vi "onPlay.vi"(8 "error in (no error)":errorcluster, 10 "Player In":refnum<class "Player.lvclass">, 11 "ReadyState in":refnum<class "ReadyState.lvclass">) -> (0 "error out":errorcluster, 1 "String":string, 2 "Player Out":refnum<class "Player.lvclass">, 3 "ReadyState out":refnum<class "ReadyState.lvclass">)   [LabVIEW 2018, in "ReadyState.lvclass"]
uses:
  ReadyState.lvclass
  Player Class/Player.lvclass
  PlayingState Class/PlayingState.lvclass
  C:/Users/fflores/Documents/LabVIEW-Open-Projects/LabIVEW OOP Design Patterns/State Pattern/State Class/State.lvclass
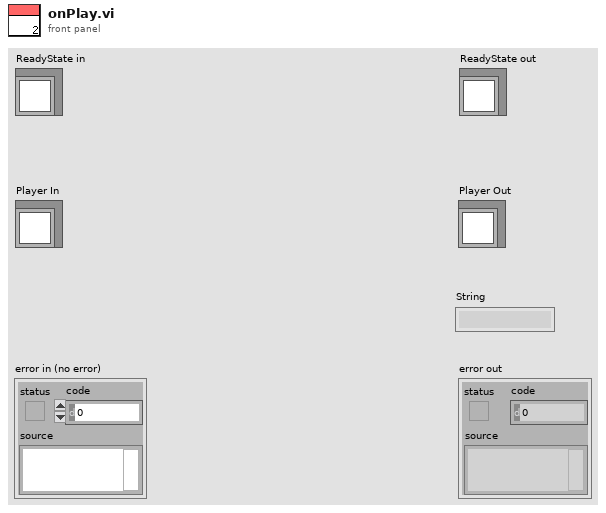
[diagram p1: front panel]
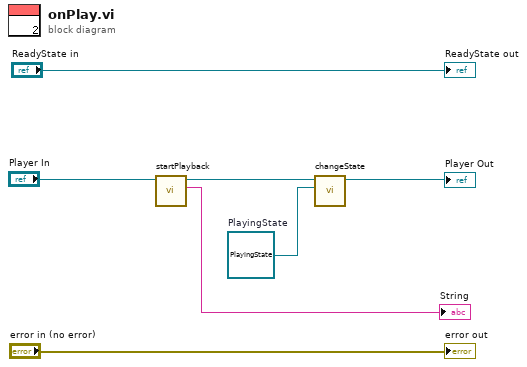
[diagram p0: block diagram]
diagram:
  w3 = refnum<class "PlayingState.lvclass"> refnum  # PlayingState
  n1 = call "startPlayback.vi"("Player in"="Player In") -> ("Song"=→"String":string, "Player out"=w2:refnum<class "Player.lvclass">)  [unwired: 8 in, 1 out]
  n2 = call-dynamic "changeState.vi"("State"=w3, "Player in"=w2) -> ("Player out"=→"Player Out":refnum<class "Player.lvclass">)  [unwired: 8 in, 1 out]
  "error out" <- "error in (no error)"
  "ReadyState out" <- "ReadyState in"
